vi "SetCellColorByString.vi"(6 "Value":u32(colorbox), 7 "WorkSheetName":string, 8 "error in (no error)":errorcluster, 9 "Column Index":i32, 10 "Row Index":i32, 11 "ExcelFile in":refnum<class "PortableExcelFileManipulationOXML.lvclass">) -> (0 "error out":errorcluster, 3 "ExcelFile out":refnum<class "PortableExcelFileManipulationOXML.lvclass">)   [LabVIEW 2019, in "PortableExcelFileManipulationOXML.lvclass"]
doc: "Sets A Cell value on an excel spreadsheet, The inputs allow the value to be input as string or a number. It also allows the worksheet index to be chosen."
uses:
  PortableExcelFileManipulationOXML.lvclass
  PortableExcelFileManipulationOXML.lvclass/PortableExcelFileManipulationOXML.ctl
  H:/LV projects/ExpressionEvaluator/Excel/ExcelManipulation.dll
  ExcelManipulation.dll
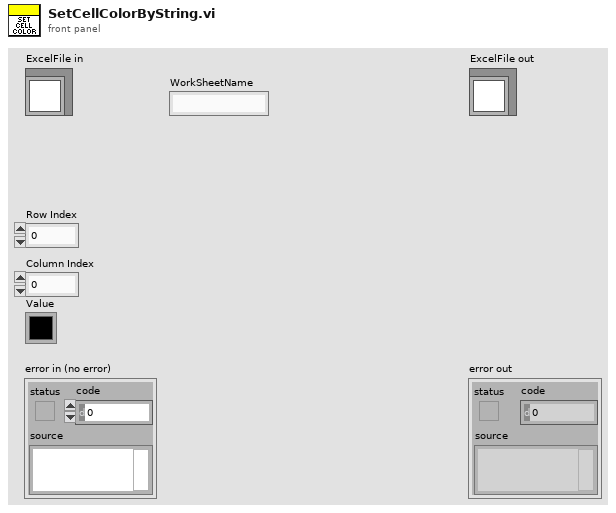
[diagram p1: front panel]
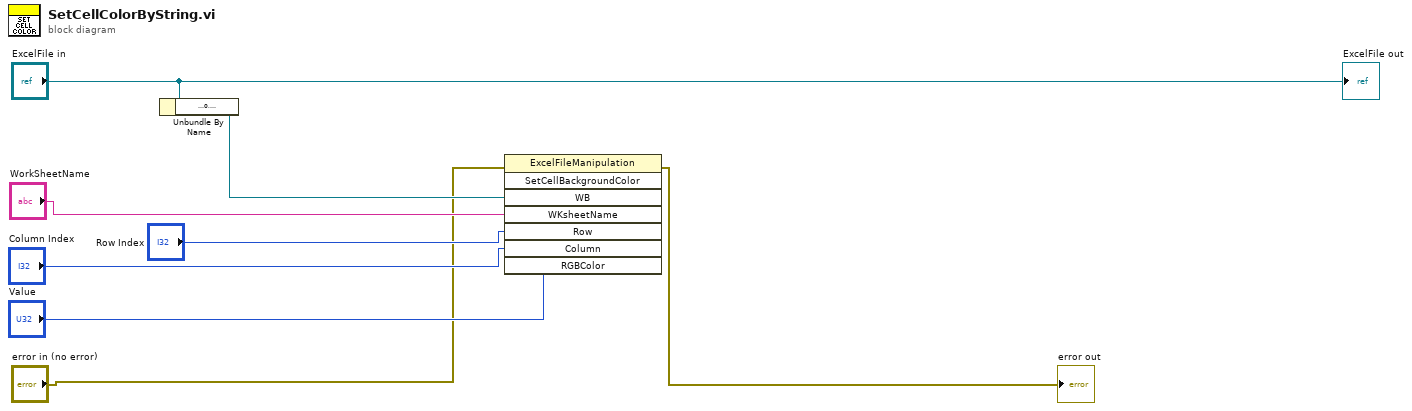
[diagram p0: block diagram]
diagram:
  n1 = Unbundle By Name("ExcelFile in") -> ("ExcelOpen"=w7:refnum<k24>)
  n2 = invoke class="ExcelFileManipulation" method="SetCellBackgroundColor"(error in="error in (no error)", "WB"=w7, "WKsheetName"="WorkSheetName", "Row"="Row Index", "Column"="Column Index", "RGBColor"="Value") -> (error out=→"error out":errorcluster)  [unwired: 2 in, 7 out]
  "ExcelFile out" <- "ExcelFile in"
